vi "MovingAverage.vi"(3 "error in":errorcluster, 4 "Points to average":i32=200, 5 "Input array":dbl[](array[numeric])) -> (0 "error out":errorcluster, 2 "Output array":dbl[](array[numeric]))   [LabVIEW 2014]
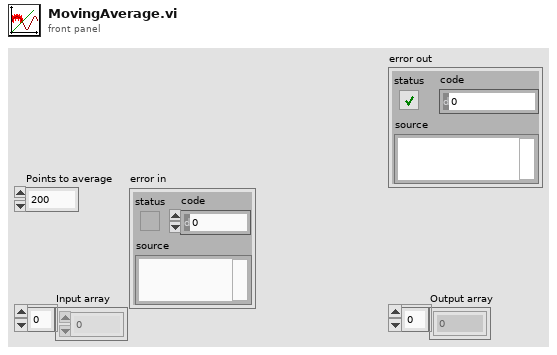
[diagram p1: front panel]
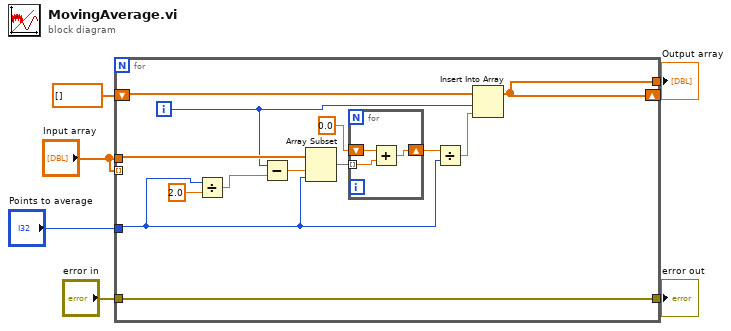
[diagram p0: block diagram]
diagram:
  n1 = for {
    tunnel: [w15] -> w5
    shift-right: [w15] -> _
    shift-left: dbl[] [] -> [w14]
    tunnel: "Input array" -> [_] mode=indexing
    tunnel: "Input array" -> [w13]
    tunnel: "Points to average" -> [w10]
    tunnel: "error in" -> [w12]
    tunnel: [w12] -> w1
    i -> [w8]
    n2 = Divide(x=w10, y=2.0) -> (x/y=w7:dbl)
    n3 = Subtract(x=w8, y=w7) -> (x-y=w9:dbl)
    n4 = Array Subset(array=w13, index=w9, length=w10) -> (w19:dbl[])
    n5 = for {
      tunnel: w19 -> [w20] mode=indexing
      shift-right: [w22] -> w17
      shift-left: 0.0 -> [w21]
      n6 = Add(x=w21, y=w20) -> (x+y=w22:dbl)
    }
    n7 = Divide(x=w17, y=w10) -> (x/y=w16:dbl)
    n8 = Insert Into Array(array=w14, index=w8, new element=w16) -> (w15:dbl[])
  }
  "Output array" <- w5
  "error out" <- w1
